vi "Convert HSB.vi"(10 "HSB":T1) -> (2 "Hue Sat Bri":T2)   [LabVIEW 2020, in "LMH-Hue.lvlib"]
uses:
  LMH-Hue.lvlib
  Type Defs/JSON/Hue Sat Bri.ctl
  Type Defs/HSB.ctl
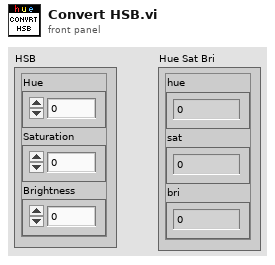
[diagram p1: front panel]
types:
  T1 = typedef "LMH-Hue.lvlib/HSB.ctl" = cluster{"Hue":u16, "Saturation":u8, "Brightness":u8}
  T2 = typedef "LMH-Hue.lvlib/Hue Sat Bri.ctl" = cluster{"hue":u16, "sat":u8, "bri":u8}
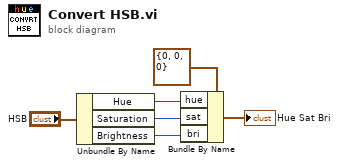
[diagram p0: block diagram]
diagram:
  n1 = Unbundle By Name("HSB") -> ("Hue"=w1:u16, "Saturation"=w2:u8, "Brightness"=w3:u8)
  n2 = Bundle By Name(cluster=T2 {"hue"=0, "sat"=0, "bri"=0} ("Hue Sat Bri"), "hue"=w1, "sat"=w2, "bri"=w3) -> (→"Hue Sat Bri":T2)
